vi "Teleop.vi"(10 "Match Info":T4={"Autonomous Elapsed Seconds"=0.0, "TeleOp Elapsed Seconds"=0.0, "Disabled Elapsed Seconds"=0.0, "Visited Autonomous"=FALSE, "Visited TeleOp"=FALSE, "Visited Disabled"=FALSE, "Autonomous Settings"={"Autonomous Style"=enum."Independent", "VI Refnum"=refnum}}, 11 "Call Context":T5) -> ()   [LabVIEW 2015]
doc: "This VI is called for each TeleOp packet received from the DS where the robot is not disabled. It is often used to read from the joysticks and update I/O or to update setpoints for timed control loops. It should complete and return within 20 milliseconds or it may miss DS packets."
uses:
  <vilib>/Rock Robotics/WPI/DriverStation/WPI_DriverStationDerivedRobotMode.ctl
  <vilib>/Rock Robotics/WPI/DriverStation/WPI_DriverStationMatch Info.ctl
  <vilib>/Rock Robotics/WPI/CAN/TalonSRX/WPI_CANTalonSRX_GlobalStatus.ctl
  <vilib>/Rock Robotics/WPI/Solenoid/WPI_SolenoidValue.ctl
  <vilib>/Rock Robotics/WPI/CAN/TalonSRX/WPI_CANTalonSRX_APIFeedbackSelect.ctl
  <vilib>/Rock Robotics/WPI/CAN/TalonSRX/WPI_CANTalonSRX_APIControlMode.ctl
  <vilib>/Rock Robotics/WPI/CAN/TalonSRX/WPI_CANTalonSRX_BrakeOverride.ctl
  <vilib>/Rock Robotics/WPI/Solenoid/WPI_SolenoidGetEnum.vi
  <vilib>/Rock Robotics/WPI/Utilities/WPI_GetSetVariantRefNum.vi
  <vilib>/Rock Robotics/Network Tables/NT Write Boolean Array.vi
  <vilib>/Rock Robotics/Network Tables/NT Write Numeric Array.vi
  <vilib>/Rock Robotics/WPI/Solenoid/WPI_SolenoidSetEnum.vi
  <vilib>/addons/control/pid/pid.llb/PID (DBL).vi
  <vilib>/Rock Robotics/Network Tables/NT Write Boolean.vi
  ADIS16448/ADI MXP IMU/FRC_ADIS16448_IMU.lvlib
  <vilib>/addons/control/pid/NI_PID_pid.lvlib
  Robot Global Data.vi
panel:
  out "Straight Line PID":dbl(graph)
  in  "Straight Line PID gains":T1={"proportional gain (Kc)"=0.15, "integral time (Ti, min)"=0.0, "derivative time (Td, min)"=0.0005} {"proportional gain (Kc)" step=0.001; "integral time (Ti, min)" step=0.001; "derivative time (Td, min)" step=0.001}
  in  "straight line output range":cluster{"output high":dbl, "output low":dbl}={"output high"=1.0, "output low"=-1.0}
  out "SRX Status Right":T2
  in  "Ramp Rate":dbl format="%#_13g"
  in  "I Zone":dbl format="%#_13g"
  in  "F":dbl=0.005212 format="%#_13g"
  in  "D":dbl format="%#_13g"
  in  "I":dbl format="%#_13g"
  in  "P":dbl=0.5 format="%#_13g"
  out "SRX Status Left":T2
  out "Override":bool
  out "Speed":T3(graph)
  # "Drive PID Tuning"
  # "Competition Robot:\n\nP = 0.5\nI = 0\nD = 0\nF = 0.005212\nI Zone = 0\nRamp Rate = 0"
  # "Competition Robot:\nOutput Range\n0.6 / -0.6\n\nP = 30\nI = 0.5\nD = 0"
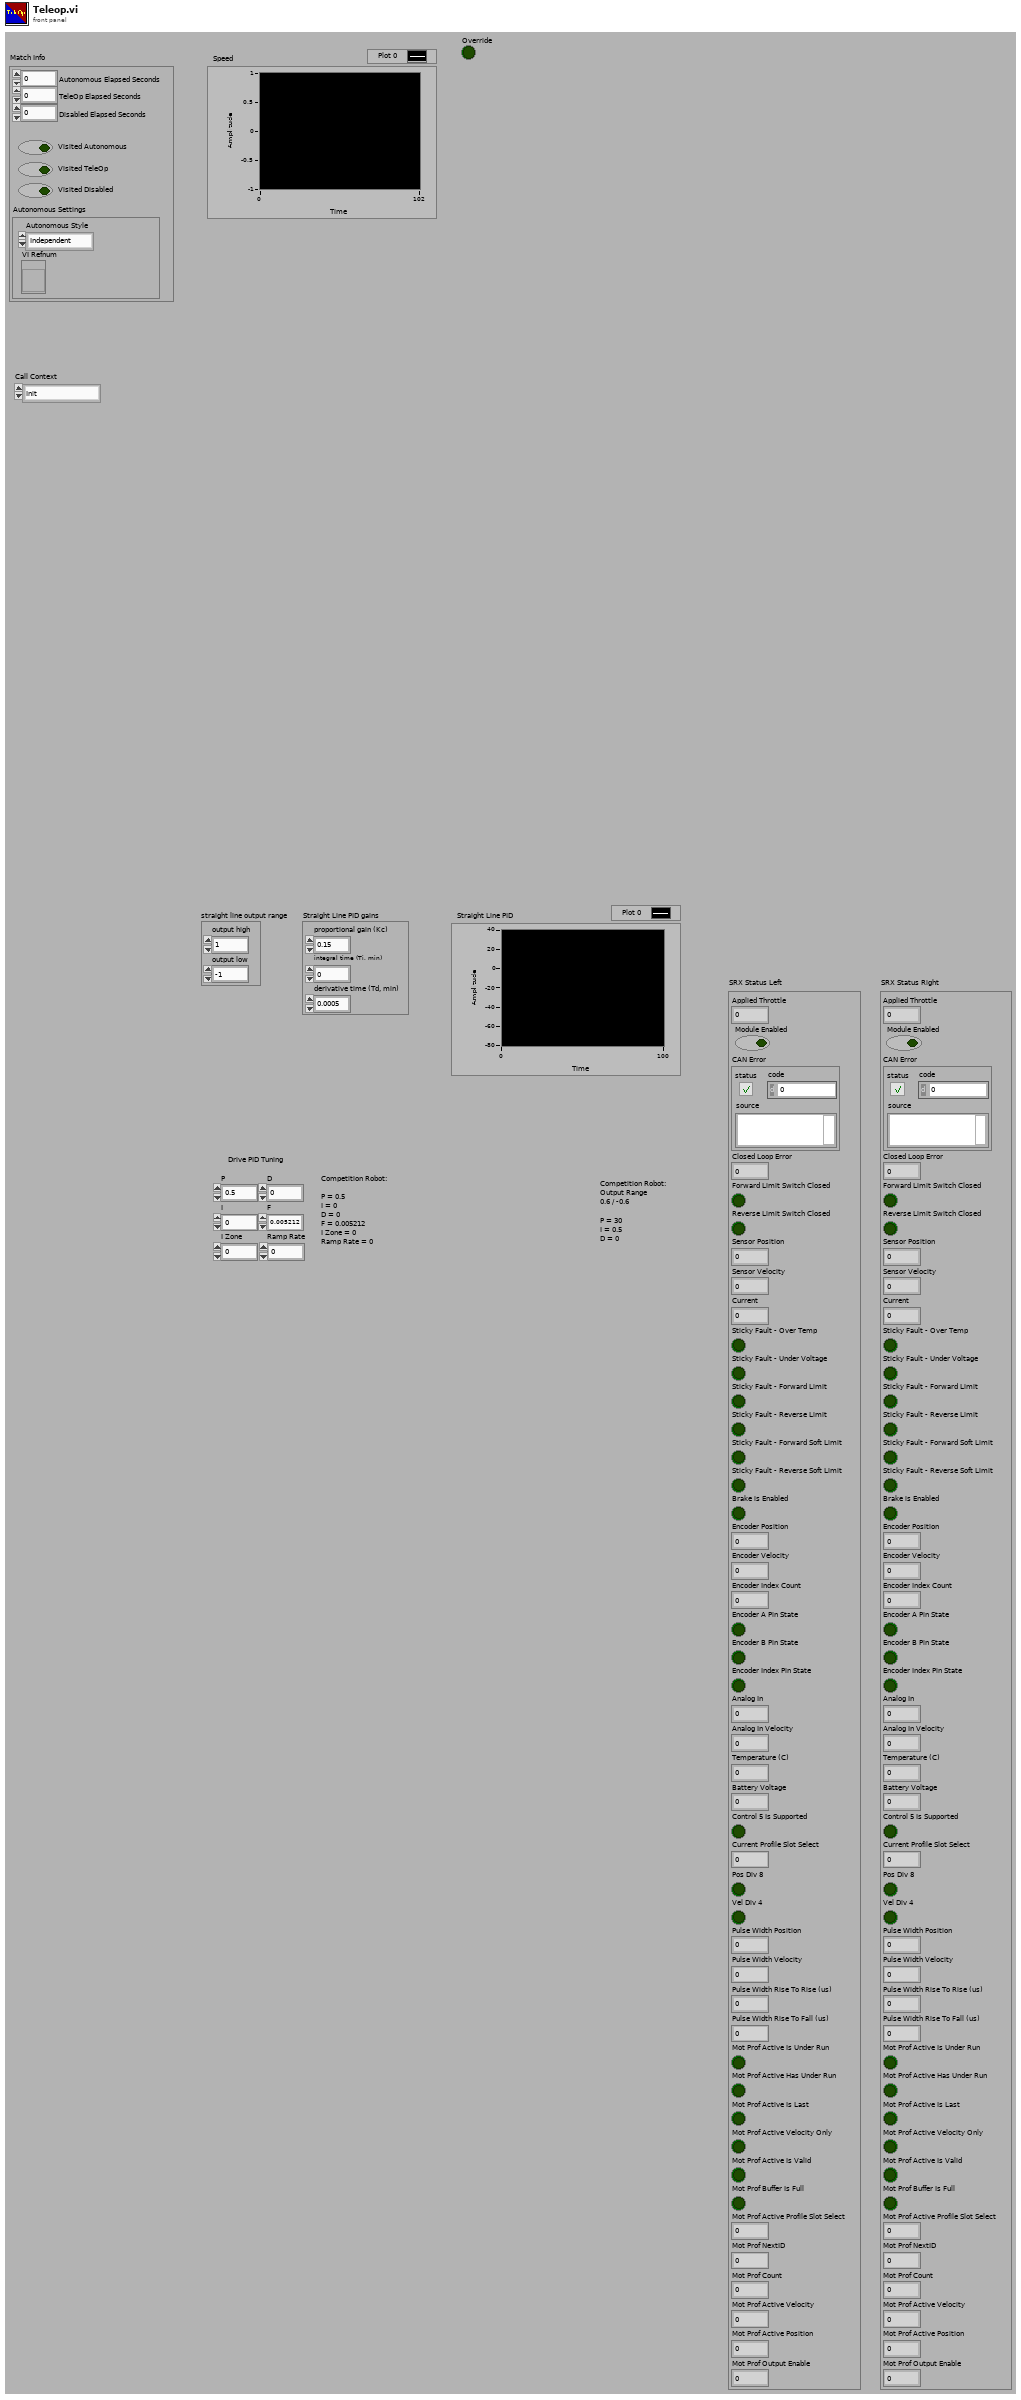
[diagram p1: front panel]
types:
  T1 = cluster{"proportional gain (Kc)":dbl, "integral time (Ti, min)":dbl, "derivative time (Td, min)":dbl}
  T2 = typedef "WPI_CANTalonSRX_GlobalStatus.ctl" = cluster{"Applied Throttle":dbl, "Module Enabled":bool, "CAN Error":errorcluster, "Closed Loop Error":dbl, "Forward Limit Switch Closed":bool, "Reverse Limit Switch Closed":bool, "Sensor Position":dbl, "Sensor Velocity":dbl, "Current":dbl, "Sticky Fault - Over Temp":bool, "Sticky Fault - Under Voltage":bool, "Sticky Fault - Forward Limit":bool, "Sticky Fault - Reverse Limit":bool, "Sticky Fault - Forward Soft Limit":bool, "Sticky Fault - Reverse Soft Limit":bool, "Brake is Enabled":bool, "Encoder Position":dbl, "Encoder Velocity":dbl, "Encoder Index Count":dbl, "Encoder A Pin State":bool, "Encoder B Pin State":bool, "Encoder Index Pin State":bool, "Analog In":dbl, "Analog In Velocity":dbl, "Temperature (C)":dbl, "Battery Voltage":dbl, "Control 5 Is Supported":bool, "Current Profile Slot Select":dbl, "Pos Div 8":bool, "Vel Div 4":bool, "Pulse Width Position":i32, "Pulse Width Velocity":i32, "Pulse Width Rise To Rise (us)":i32, "Pulse Width Rise To Fall (us)":i32, "Mot Prof Active Is Under Run":bool, "Mot Prof Active Has Under Run":bool, "Mot Prof Active Is Last":bool, "Mot Prof Active Velocity Only":bool, "Mot Prof Active Is Valid":bool, "Mot Prof Buffer Is Full":bool, "Mot Prof Active Profile Slot Select":i32, "Mot Prof NextID":i32, "Mot Prof Count":i32, "Mot Prof Active Velocity":dbl, "Mot Prof Active Position":dbl, "Mot Prof Output Enable":i32}
  T3 = cluster{"Left Motor Value":dbl, "Right Motor Value":dbl}
  T4 = typedef "WPI_DriverStationMatch Info.ctl" = cluster{"Autonomous Elapsed Seconds":dbl, "TeleOp Elapsed Seconds":dbl, "Disabled Elapsed Seconds":dbl, "Visited Autonomous":bool, "Visited TeleOp":bool, "Visited Disabled":bool, "Autonomous Settings":cluster{"Autonomous Style":enum16{"Iterative", "Independent"}, "VI Refnum":refnum<vi>}}
  T5 = typedef "WPI_DriverStationDerivedRobotMode.ctl" = enum16{"Init", "Execute", "Stop"}
  T6 = typedef "WPI_SolenoidValue.ctl" = enum16{"Off", "On", "Forward", "Reverse"}
  T7 = typedef "WPI_MotorControlDeviceRef.ctl" = cluster{"DeviceStatus":errorcluster, "Type":T8, "PWM":cluster{"PWM Channel":T9, "DeadBand":T10}, "CAN":cluster{"Device Number":u8, "Control Mode":T11, "Semaphore":T12, "Max Vout":dbl, "TalonSRX Control Mode":T13}, "Invert":bool}
  T8 = typedef "WPI_MotorControlType.ctl" = enum16{"PWM", "CAN", "CANTalonSRX"}
  T9 = typedef "FPGA_DIOPWMChannel.ctl" = enum8{"PWM 0", "PWM 1", "PWM 2", "PWM 3", "PWM 4", "PWM 5", "PWM 6", "PWM 7", "PWM 8", "PWM 9", "PWM MXP 0", "PWM MXP 1", "PWM MXP 2", "PWM MXP 3", "PWM MXP 4", "PWM MXP 5", "PWM MXP 6", "PWM MXP 7", "PWM MXP 8", "PWM MXP 9", "Invalid"}
  T10 = typedef "WPI_PWMDeadband.ctl" = cluster{"Name":string, "maxPositivePwm":i32, "minPositivePwm":i32, "centerPwm":i32, "maxNegativePwm":i32, "minNegativePwm":i32, "angularRange":u16}
  T11 = typedef "WPI_CANJaguar_ControlMode.ctl" = enum8{"Percent VBus", "Current", "Speed", "Position", "Voltage"}
  T12 = typedef "Semaphore RefNum" = refnum<k1>
  T13 = typedef "WPI_CANTalonSRX_APIControlMode.ctl" = enum8{"Percent VBus", "Speed", "Position", "Slave", "Unchanged / Invalid", "Voltage Compensation", "Current", "Motion Profile"}
  T14 = typedef "WPI_JoystickDevRef.ctl" = cluster{"Device":T15}
  T15 = typedef "WPI_JoystickDeviceEnum.ctl" = enum16{"USB 0", "USB 1", "USB 2", "USB 3", "USB 4", "USB 5"}
  T16 = typedef "WPI_SolenoidDevRef.ctl" = cluster{"DevStatus":errorcluster, "Pneumatics Control Module":u8, "Forward Solenoid Channel":T17, "Reverse Solenoid Channel":T17}
  T17 = typedef "WPI_SolenoidChannel.ctl" = enum8{"Solenoid 0", "Solenoid 1", "Solenoid 2", "Solenoid 3", "Solenoid 4", "Solenoid 5", "Solenoid 6", "Solenoid 7", "Invalid"}
  T18 = typedef "WPI_SwitchDevRef.ctl" = cluster{"DevStatus":errorcluster, "DIO Channel":T19, "CntIndex":T20, "Normally Closed":bool}
  T19 = typedef "FPGA_DIOChannel.ctl" = enum8{"DIO 0", "DIO 1", "DIO 2", "DIO 3", "DIO 4", "DIO 5", "DIO 6", "DIO 7", "DIO 8", "DIO 9", "DIO MXP 0", "DIO MXP 1", "DIO MXP 2", "DIO MXP 3", "DIO MXP 4", "DIO MXP 5", "DIO MXP 6", "DIO MXP 7", "DIO MXP 8", "DIO MXP 9", "DIO MXP 10", "DIO MXP 11", "DIO MXP 12", "DIO MXP 13", "DIO MXP 14", "DIO MXP 15", "Invalid"}
  T20 = typedef "FPGA_CounterCtrSystemIndex.ctl" = enum8{"Ctr 0", "Ctr 1", "Ctr 2", "Ctr 3", "Ctr 4", "Ctr 5", "Ctr 6", "Ctr 7", "Invalid"}
  T21 = typedef "FRC_ADIS16448_IMU.lvlib/WPI_IMU_ADIS16448_InterruptDevRef.ctl" = cluster{"ADI IMU DevRef":T22, "InterruptRef":T24}
  T22 = typedef "FRC_ADIS16448_IMU.lvlib/WPI_IMU_ADIS16448_IMUDevRef.ctl" = cluster{"DevStatus":errorcluster, "Handle":i32, "SPI Bus":T23, "Device Found":bool, "Device Ready":bool, "Yaw Axis":enum16{"X", "Y", "Z"}, "AHRS Algorithm":enum16{"Complementary", "Madgwick"}, "Serial":u16, "Lot ID 2":u16, "Lot ID 1":u16, "Product ID":u16}
  T23 = typedef "spi_bus.ctl" = enum16{"SPI On-Board, CS0", "SPI On-Board, CS1", "SPI On-Board, CS2", "SPI On-Board, CS3", "SPI MXP", "Invalid"}
  T24 = typedef "WPI_InterruptRef.ctl" = cluster{"DevStatus":errorcluster, "InterruptIndex":T25}
  T25 = typedef "FPGA_InterruptIndex.ctl" = enum8{"0", "1", "2", "3", "4", "5", "6", "7", "Invalid"}
  T26 = cluster{"X Angle":dbl, "Y Angle":dbl, "Z Angle":dbl}
  T27 = typedef "WPI_CANTalonSRX_APIFeedbackSelect.ctl" = enum16{"Digital Quadrature Encoder", "Analog Potentiometer", "Analog Encoder", "Count on Quad-A (Rising-Edge)", "Count on Quad-A (Falling-Edge)", "CTR Magnetic Enc (Absolute)", "CTR Magnetic Enc (Relative)", "Pulse Width"}
  T28 = typedef "WPI_CANTalonSRX_BrakeOverride.ctl" = enum8{"No Override", "Override to Coast", "Override to Brake"}
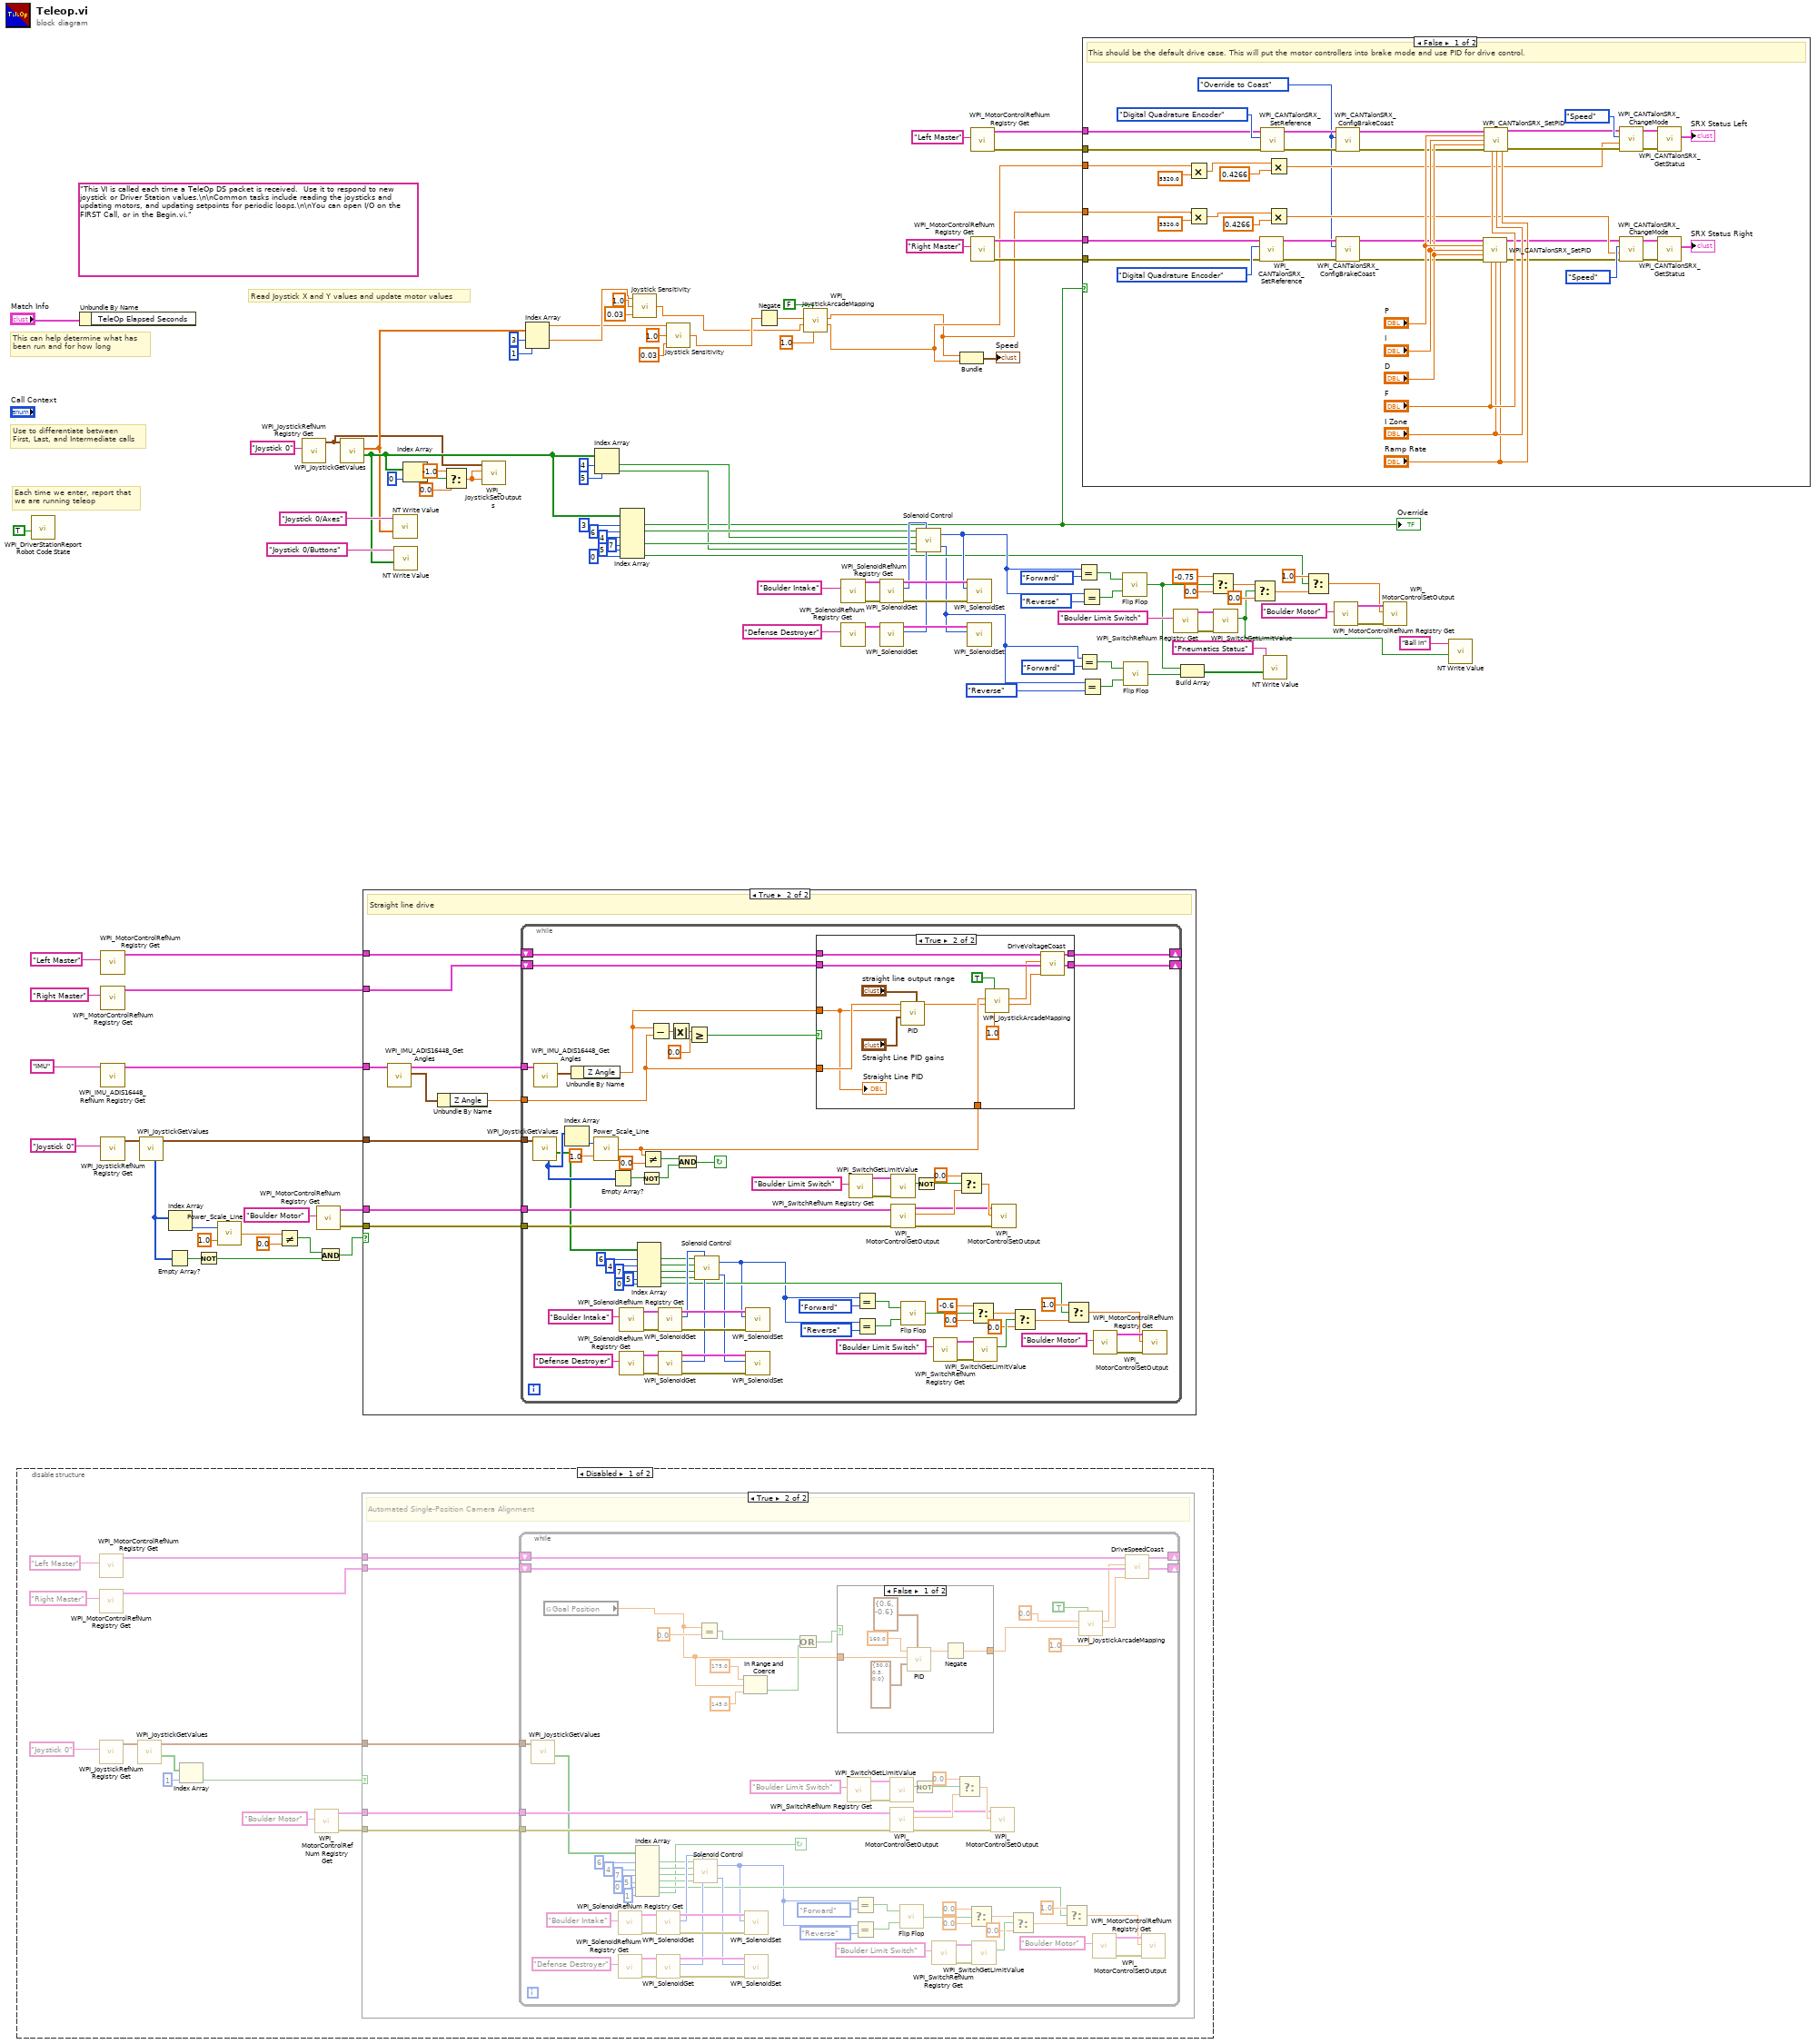
[diagram p0: block diagram]
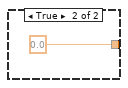
[diagram p3: hidden frame]
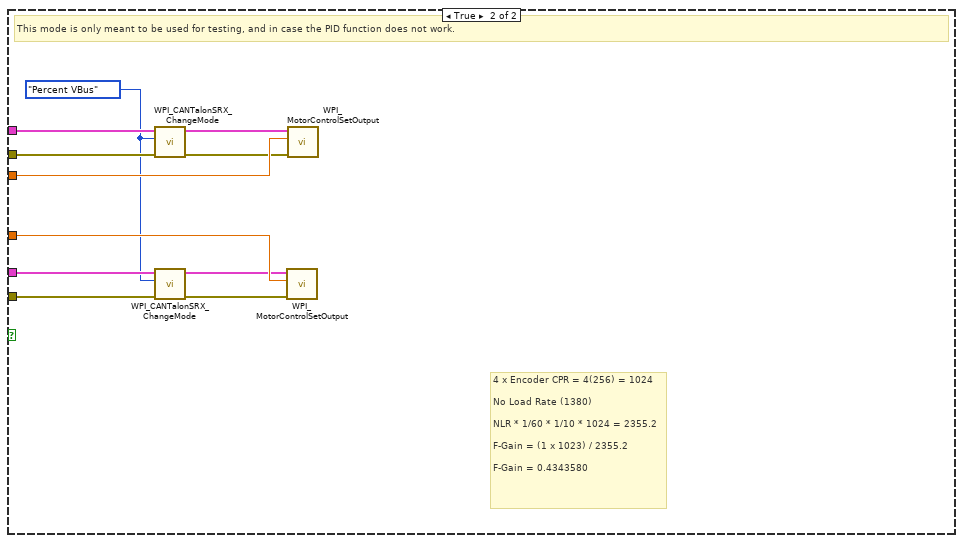
[diagram p5: hidden frame]
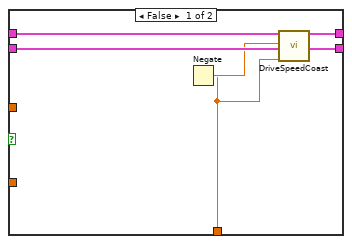
[diagram p7: hidden frame]
diagram:
  (unwired) "This VI is called each time a TeleOp DS packet is received.  Use it to respond to new joystick or Driver Station values.\n\nCommon tasks include reading the joysticks and updating motors, and updating setpoints for periodic loops.\n\nYou can open I/O on the FIRST Call, or in the Begin.vi."
  # "Each time we enter, report that\nwe are running teleop"
  # "Use to differentiate between\nFirst, Last, and Intermediate calls"
  # "This can help determine what has\nbeen run and for how long"
  # "Read Joystick X and Y values and update motor values"
  n1 = disable-structure shown="Disabled" {
    frame Disabled {
      n2 = call <vilib>:"WPI_MotorControlRefNum Registry Get.vi"("refnum name"="Left Master") -> ("MotorControlDevRef"=w111:T7)  [unwired: 9 in, 1 out]
      n3 = call <vilib>:"WPI_MotorControlRefNum Registry Get.vi"("refnum name"="Right Master") -> ("MotorControlDevRef"=w110:T7)  [unwired: 9 in, 1 out]
      n4 = call <vilib>:"WPI_JoystickRefNum Registry Get.vi"("refnum name"="Joystick 0") -> ("JoystickDevRef"=w119:T14)  [unwired: 1 in, 9 out]
      n5 = call <vilib>:"WPI_JoystickGetValues.vi"("JoystickDevRef"=w119) -> ("Buttons"=w114:bool[], "JoystickDevRef"=w118:T14)  [unwired: 6 in, 3 out]
      n6 = Index Array(array=w114, index=1) -> (element=w112:bool)
      n7 = call <vilib>:"WPI_MotorControlRefNum Registry Get.vi"("refnum name"="Boulder Motor") -> ("error out"=w115:errorcluster, "MotorControlDevRef"=w116:T7)  [unwired: 9 in]
      n8 = case shown="True" w112 {
        tunnel: w110 -> [_ w127]
        tunnel: w111 -> [_ w126]
        tunnel: w118 -> [_ w125]
        tunnel: w116 -> [_ w124]
        tunnel: w115 -> [_ w123]
        frame False {
          # "POV not pressed"
        }
        frame True {
          # "Automated Single-Position Camera Alignment"
          n9 = while {
            shift-right: [w202] -> _
            shift-left: w127 -> [w201]
            shift-right: [w203] -> _
            shift-left: w126 -> [w200]
            tunnel: w125 -> [w199]
            tunnel: w124 -> [w191]
            tunnel: w123 -> [w190]
            stop <- w137 continue-if-true
            n10 = call <vilib>:"WPI_JoystickGetValues.vi"("JoystickDevRef"=w199) -> ("Buttons"=w145:bool[])  [unwired: 6 in, 4 out]
            n11 = global read "Robot Global Data.vi" "Goal Position"() -> (w128:dbl)
            n12 = call <vilib>:"WPI_SolenoidRefNum Registry Get.vi"("refnum name"="Boulder Intake") -> ("error out"=w162:errorcluster, "SolenoidDevRef"=w165:T16)  [unwired: 9 in]
            n13 = call <vilib>:"WPI_SolenoidRefNum Registry Get.vi"("refnum name"="Defense Destroyer") -> ("error out"=w160:errorcluster, "SolenoidDevRef"=w161:T16)  [unwired: 9 in]
            n14 = Index Array(array=w145, index #1=6 ("index"), index #2=4 ("index"), index #3=7 ("index"), index #4=5 ("index"), index #5=0 ("index"), index #6=1 ("index")) -> (element #1=w150:bool, element #2=w149:bool, element #3=w148:bool, element #4=w147:bool, element #5=w146:bool, element #6=w137:bool)
            n15 = call-poly <vilib>:"WPI_SolenoidGet.vi"("error in (no error)"=w162, "SolenoidDevRef"=w165) -> ("error out"=w163:errorcluster, "Value"=w157:T6, "SolenoidDevRef"=w164:T16)  [unwired: 7 in]
            n16 = call-poly <vilib>:"WPI_SolenoidGet.vi"("error in (no error)"=w160, "SolenoidDevRef"=w161) -> ("error out"=w158:errorcluster, "Value"=w156:T6, "SolenoidDevRef"=w159:T16)  [unwired: 7 in]
            n17 = call "Solenoid Control.vi"("Defense Get"=w156, "Ball Get"=w157, "Both Down"=w147, "Both Up"=w148, "Ball Down"=w149, "Ball Up"=w150) -> ("Defense Output"=w155:T6, "Ball Output"=w144:T6)
            n18 = Equal?(x=w128, y=0.0) -> (x = y?=w131:bool)
            n19 = In Range and Coerce(upper limit=175.0, x=w128, lower limit=145.0) -> (In Range?=w130:bool)  [unwired: 1 out]
            n20 = call-poly <vilib>:"WPI_SolenoidSet.vi"("error in (no error)"=w163, "Value"=w144, "SolenoidDevRef"=w164) -> ()  [unwired: 7 in, 2 out]
            n21 = call-poly <vilib>:"WPI_SolenoidSet.vi"("error in (no error)"=w158, "Value"=w155, "SolenoidDevRef"=w159) -> ()  [unwired: 7 in, 2 out]
            n22 = Or(x=w131, y=w130) -> (x .or. y?=w132:bool)
            n23 = case shown="False" w132 {
              tunnel: w128 -> [w209 _]
              tunnel: [w207 0.0 ("output")] -> w135
              frame False {
                n24 = call-poly <vilib>:"PID.vi"("output range"=cluster{"output high":dbl, "output low":dbl} {"output high"=0.6, "output low"=-0.6}, "PID gains"=T1 {"proportional gain (Kc)"=30.0, "integral time (Ti, min)"=0.5, "derivative time (Td, min)"=0.0}, "process variable"=w209, "setpoint"=160.0) -> ("output"=w208:dbl)  [unwired: 6 in, 1 out]
                n25 = Negate(x=w208) -> (-x=w207:dbl)
              }
              frame True {
              }
            }
            n26 = call <vilib>:"WPI_SwitchRefNum Registry Get.vi"("refnum name"="Boulder Limit Switch") -> ("error out"=w198:errorcluster, "SwitchDevRef"=w197:T18)  [unwired: 9 in]
            n27 = Equal?(x=w144, y=WPI_SolenoidValue."Forward" ("Ball Output")) -> (x = y?=w153:bool)
            n28 = Equal?(x=w144, y=WPI_SolenoidValue."Reverse") -> (x = y?=w151:bool)
            n29 = call <vilib>:"WPI_SwitchGetLimitValue.vi"("error in (no error)"=w198, "SwitchDevRef"=w197) -> ("Switch Pressed"=w188:bool)  [unwired: 7 in, 2 out]
            n30 = call <vilib>:"WPI_MotorControlGetOutput.vi"("error in (no error)"=w190, "MotorControlDevRef"=w191) -> ("error out"=w192:errorcluster, "Output"=w194:dbl, "MotorControlDevRef"=w193:T7)  [unwired: 7 in]
            n31 = call "Flip Flop.vi"("Reset"=w151, "Value to be latched"=w153) -> ("Indicator"=w169:bool)
            n32 = Not(x=w188) -> (.not. x?=w189:bool)
            n33 = call <vilib>:"WPI_SwitchRefNum Registry Get.vi"("refnum name"="Boulder Limit Switch") -> ("error out"=w179:errorcluster, "SwitchDevRef"=w178:T18)  [unwired: 9 in]
            n34 = Select(t=0.0, s=w189, f=w194) -> (s? t:f=w195:dbl)
            n35 = Select(t=0.0, s=w169, f=0.0) -> (s? t:f=w173:dbl)
            n36 = call <vilib>:"WPI_SwitchGetLimitValue.vi"("error in (no error)"=w179, "SwitchDevRef"=w178) -> ("Switch Pressed"=w175:bool)  [unwired: 7 in, 2 out]
            n37 = call <vilib>:"WPI_MotorControlSetOutput.vi"("error in (no error)"=w192, "Output"=w195, "MotorControlDevRef"=w193) -> ()  [unwired: 6 in, 3 out]
            n38 = Select(t=w173, s=w175, f=0.0) -> (s? t:f=w172:dbl)
            n39 = Select(t=1.0, s=w146, f=w172) -> (s? t:f=w171:dbl)
            n40 = call <vilib>:"WPI_JoystickArcadeMapping.vi"("Max Output"=1.0, "Square Inputs"=TRUE, "Y axis value"=w135, "X axis value"=0.0 ("Power Input")) -> ("Right Motor Value"=w140:dbl, "Left Motor Value"=w139:dbl)  [unwired: 6 in]
            n41 = call <vilib>:"WPI_MotorControlRefNum Registry Get.vi"("refnum name"="Boulder Motor") -> ("error out"=w181:errorcluster, "MotorControlDevRef"=w182:T7)  [unwired: 9 in]
            n42 = call "DriveSpeedCoast.vi"("Left Motor"=w200, "Left Stick"=w139, "Right Motor"=w201, "Right Stick"=w140) -> ("Left Motor Out"=w203:T7, "Right Motor Out"=w202:T7)  [unwired: 10 in, 4 out]
            n43 = call <vilib>:"WPI_MotorControlSetOutput.vi"("error in (no error)"=w181, "Output"=w171, "MotorControlDevRef"=w182) -> ()  [unwired: 6 in, 3 out]
          }
        }
      }
    }
    frame Enabled {
    }
  }
  n44 = call <vilib>:"WPI_DriverStationReport Robot Code State.vi"("TeleOp"=TRUE ("Autonomous")) -> ()  [unwired: 10 in, 1 out]
  n45 = Unbundle By Name("Match Info") -> ()  [unwired: 1 out]
  n46 = call <vilib>:"WPI_MotorControlRefNum Registry Get.vi"("refnum name"="Left Master") -> ("MotorControlDevRef"=w5:T7)  [unwired: 9 in, 1 out]
  n47 = call <vilib>:"WPI_MotorControlRefNum Registry Get.vi"("refnum name"="Right Master") -> ("MotorControlDevRef"=w4:T7)  [unwired: 9 in, 1 out]
  n48 = call "WPI_IMU_ADIS16448_RefNum Registry Get.vi"("refnum name"="IMU") -> ("ADI IMU Interrupt DevRef"=w24:T21)  [unwired: 9 in, 1 out]
  n49 = call <vilib>:"WPI_JoystickRefNum Registry Get.vi"("refnum name"="Joystick 0") -> ("JoystickDevRef"=w21:T14)  [unwired: 1 in, 9 out]
  n50 = call <vilib>:"WPI_JoystickGetValues.vi"("JoystickDevRef"=w21) -> ("JoystickDevRef"=w20:T14, "POVs"=w19:i16[])  [unwired: 6 in, 3 out]
  n51 = Empty Array?(array=w19) -> (empty?=w18:bool)
  n52 = Index Array(array=w19) -> (element=w23:i16)  [unwired: 1 in]
  n53 = Not(x=w18) -> (.not. x?=w17:bool)
  n54 = call "Power_Scale_Line.vi"("Power Input"=1.0, "POV"=w23) -> ("Power Output"=w25:dbl)
  n55 = Not Equal?(x=w25, y=0.0) -> (x != y?=w16:bool)
  n56 = call <vilib>:"WPI_JoystickRefNum Registry Get.vi"("refnum name"="Joystick 0") -> ("JoystickDevRef"=w31:T14)  [unwired: 1 in, 9 out]
  n57 = call <vilib>:"WPI_MotorControlRefNum Registry Get.vi"("refnum name"="Boulder Motor") -> ("error out"=w12:errorcluster, "MotorControlDevRef"=w13:T7)  [unwired: 9 in]
  n58 = And(x=w16, y=w17) -> (x .and. y?=w15:bool)
  n59 = call <vilib>:"WPI_JoystickGetValues.vi"("JoystickDevRef"=w31) -> ("Buttons"=w38:bool[], "Axes"=w32:dbl[])  [unwired: 6 in, 3 out]
  n60 = case shown="True" w15 {
    tunnel: w24 -> [_ w211]
    tunnel: w20 -> [_ w218]
    tunnel: w13 -> [_ w215]
    tunnel: w12 -> [_ w214]
    tunnel: w5 -> [_ w213]
    tunnel: w4 -> [_ w212]
    frame False {
      # "POV not pressed"
    }
    frame True {
      # "Straight line drive"
      n61 = call "WPI_IMU_ADIS16448_Get Angles.vi"("ADI IMU Interrupt DevRef"=w211) -> ("IMU Angles Out"=w216:T26, "ADI IMU Interrupt DevRef Out"=w217:T21)  [unwired: 7 in, 2 out]
      n62 = Unbundle By Name(w216) -> ("Z Angle"=w219:dbl)
      n63 = while {
        tunnel: w217 -> [w278]
        tunnel: w219 -> [w289]
        shift-right: [w293] -> _
        shift-left: w212 -> [w292]
        shift-right: [w294] -> _
        shift-left: w213 -> [w291]
        tunnel: w218 -> [w286]
        tunnel: w215 -> [w269]
        tunnel: w214 -> [w268]
        stop <- w282 continue-if-true
        n64 = call <vilib>:"WPI_JoystickGetValues.vi"("JoystickDevRef"=w286) -> ("Buttons"=w222:bool[], "POVs"=w281:i16[])  [unwired: 6 in, 3 out]
        n65 = call "WPI_IMU_ADIS16448_Get Angles.vi"("ADI IMU Interrupt DevRef"=w278) -> ("IMU Angles Out"=w277:T26)  [unwired: 7 in, 3 out]
        n66 = Index Array(array=w281) -> (element=w295:i16)  [unwired: 1 in]
        n67 = Unbundle By Name(w277) -> ("Z Angle"=w267:dbl)
        n68 = call "Power_Scale_Line.vi"("Power Input"=1.0, "POV"=w295) -> ("Power Output"=w290:dbl)
        n69 = Empty Array?(array=w281) -> (empty?=w285:bool)
        n70 = call <vilib>:"WPI_SolenoidRefNum Registry Get.vi"("refnum name"="Boulder Intake") -> ("error out"=w239:errorcluster, "SolenoidDevRef"=w242:T16)  [unwired: 9 in]
        n71 = call <vilib>:"WPI_SolenoidRefNum Registry Get.vi"("refnum name"="Defense Destroyer") -> ("error out"=w237:errorcluster, "SolenoidDevRef"=w238:T16)  [unwired: 9 in]
        n72 = Index Array(array=w222, index #1=6 ("index"), index #2=4 ("index"), index #3=7 ("index"), index #4=5 ("index"), index #5=0 ("index")) -> (element #1=w227:bool, element #2=w226:bool, element #3=w225:bool, element #4=w224:bool, element #5=w223:bool)
        n73 = Not(x=w285) -> (.not. x?=w284:bool)
        n74 = Not Equal?(x=w290, y=0.0) -> (x != y?=w283:bool)
        n75 = Subtract(x=w267, y=w289) -> (x-y=w280:dbl)
        n76 = call-poly <vilib>:"WPI_SolenoidGet.vi"("error in (no error)"=w239, "SolenoidDevRef"=w242) -> ("error out"=w240:errorcluster, "Value"=w234:T6, "SolenoidDevRef"=w241:T16)  [unwired: 7 in]
        n77 = call-poly <vilib>:"WPI_SolenoidGet.vi"("error in (no error)"=w237, "SolenoidDevRef"=w238) -> ("error out"=w235:errorcluster, "Value"=w233:T6, "SolenoidDevRef"=w236:T16)  [unwired: 7 in]
        n78 = Absolute Value(x=w280) -> (abs(x)=w279:dbl)
        n79 = And(x=w283, y=w284) -> (x .and. y?=w282:bool)
        n80 = Greater Or Equal?(x=w279, y=0.0 ("within")) -> (x >= y?=w287:bool)
        n81 = call "Solenoid Control.vi"("Defense Get"=w233, "Ball Get"=w234, "Both Down"=w224, "Both Up"=w225, "Ball Down"=w226, "Ball Up"=w227) -> ("Defense Output"=w232:T6, "Ball Output"=w221:T6)
        n82 = call-poly <vilib>:"WPI_SolenoidSet.vi"("error in (no error)"=w240, "Value"=w221, "SolenoidDevRef"=w241) -> ()  [unwired: 7 in, 2 out]
        n83 = call-poly <vilib>:"WPI_SolenoidSet.vi"("error in (no error)"=w235, "Value"=w232, "SolenoidDevRef"=w236) -> ()  [unwired: 7 in, 2 out]
        n84 = case shown="True" w287 {
          tunnel: [w302 w308] -> w294
          tunnel: [w301 w309] -> w293
          tunnel: w292 -> [w300 w311]
          tunnel: w291 -> [w303 w312]
          tunnel: w290 -> [w298 w306]
          tunnel: w267 -> [_ w304]
          tunnel: w289 -> [_ w317]
          frame False {
            n85 = Negate(x=w298) -> (-x=w299:dbl)
            n86 = call "DriveSpeedCoast.vi"("Left Motor"=w303, "Left Stick"=w299, "Right Motor"=w300, "Right Stick"=w298) -> ("Left Motor Out"=w302:T7, "Right Motor Out"=w301:T7)  [unwired: 10 in, 4 out]
          }
          frame True {
            n87 = call-poly <vilib>:"PID.vi"("output range"="straight line output range", "PID gains"="Straight Line PID gains", "process variable"=w304, "setpoint"=w317) -> ("output"=w305:dbl)  [unwired: 6 in, 1 out]
            n88 = call <vilib>:"WPI_JoystickArcadeMapping.vi"("Max Output"=1.0, "Square Inputs"=TRUE, "Y axis value"=w305, "X axis value"=w306) -> ("Right Motor Value"=w310:dbl, "Left Motor Value"=w307:dbl)  [unwired: 6 in]
            n89 = call "DriveVoltageCoast.vi"("Left Motor"=w312, "Left Stick"=w307, "Right Motor"=w311, "Right Stick"=w310) -> ("Left Motor Out"=w308:T7, "Right Motor Out"=w309:T7)  [unwired: 12 in, 2 out]
            "Straight Line PID" <- w304
          }
        }
        n90 = call <vilib>:"WPI_SwitchRefNum Registry Get.vi"("refnum name"="Boulder Limit Switch") -> ("error out"=w276:errorcluster, "SwitchDevRef"=w275:T18)  [unwired: 9 in]
        n91 = Equal?(x=w221, y=WPI_SolenoidValue."Forward" ("Ball Output")) -> (x = y?=w230:bool)
        n92 = Equal?(x=w221, y=WPI_SolenoidValue."Reverse") -> (x = y?=w228:bool)
        n93 = call <vilib>:"WPI_SwitchGetLimitValue.vi"("error in (no error)"=w276, "SwitchDevRef"=w275) -> ("Switch Pressed"=w265:bool)  [unwired: 7 in, 2 out]
        n94 = call <vilib>:"WPI_MotorControlGetOutput.vi"("error in (no error)"=w268, "MotorControlDevRef"=w269) -> ("error out"=w270:errorcluster, "Output"=w272:dbl, "MotorControlDevRef"=w271:T7)  [unwired: 7 in]
        n95 = call "Flip Flop.vi"("Reset"=w228, "Value to be latched"=w230) -> ("Indicator"=w246:bool)
        n96 = Not(x=w265) -> (.not. x?=w266:bool)
        n97 = call <vilib>:"WPI_SwitchRefNum Registry Get.vi"("refnum name"="Boulder Limit Switch") -> ("error out"=w256:errorcluster, "SwitchDevRef"=w255:T18)  [unwired: 9 in]
        n98 = Select(t=0.0, s=w266, f=w272) -> (s? t:f=w273:dbl)
        n99 = Select(t=-0.6, s=w246, f=0.0) -> (s? t:f=w250:dbl)
        n100 = call <vilib>:"WPI_SwitchGetLimitValue.vi"("error in (no error)"=w256, "SwitchDevRef"=w255) -> ("Switch Pressed"=w252:bool)  [unwired: 7 in, 2 out]
        n101 = call <vilib>:"WPI_MotorControlSetOutput.vi"("error in (no error)"=w270, "Output"=w273, "MotorControlDevRef"=w271) -> ()  [unwired: 6 in, 3 out]
        n102 = Select(t=w250, s=w252, f=0.0) -> (s? t:f=w249:dbl)
        n103 = Select(t=1.0, s=w223, f=w249) -> (s? t:f=w248:dbl)
        n104 = call <vilib>:"WPI_MotorControlRefNum Registry Get.vi"("refnum name"="Boulder Motor") -> ("error out"=w258:errorcluster, "MotorControlDevRef"=w259:T7)  [unwired: 9 in]
        n105 = call <vilib>:"WPI_MotorControlSetOutput.vi"("error in (no error)"=w258, "Output"=w248, "MotorControlDevRef"=w259) -> ()  [unwired: 6 in, 3 out]
      }
    }
  }
  n106 = call-poly <vilib>:"NT Write Value.vi"("Numeric Array"=w32, "Name"="Joystick 0/Axes") -> ()  [unwired: 9 in, 1 out]
  n107 = call-poly <vilib>:"NT Write Value.vi"("Boolean Array"=w38, "Name"="Joystick 0/Buttons") -> ()  [unwired: 9 in, 1 out]
  n108 = Index Array(array=w38, index=0) -> (element=w36:bool)
  n109 = Select(t=-1.0, s=w36, f=0.0) -> (s? t:f=w33:dbl)
  n110 = call <vilib>:"WPI_JoystickSetOutputs.vi"("Right Rumble"=w33, "Left Rumble"=w33, "JoystickDevRef"=w31) -> ()  [unwired: 7 in, 2 out]
  n111 = Index Array(array=w32, index #1=3 ("index"), index #2=1 ("index")) -> (element #1=w44:dbl, element #2=w43:dbl)
  n112 = Index Array(array=w38, index #1=4 ("index"), index #2=5 ("index")) -> (element #1=w55:bool, element #2=w54:bool)
  n113 = Index Array(array=w38, index #1=3 ("index"), index #2=6 ("index"), index #3=4 ("index"), index #4=7 ("index"), index #5=5 ("index"), index #6=0 ("index")) -> (element #1=w3:bool, element #2=w70:bool, element #4=w69:bool, element #6=w68:bool)  [unwired: 2 out]
  "Override" <- w3
  n114 = call "Joystick Sensitivity.vi"("B"=0.03, "A"=1.0, "X"=w44) -> ("Y"=w41:dbl)
  n115 = call "Joystick Sensitivity.vi"("B"=0.03, "A"=1.0, "X"=w43) -> ("Y"=w42:dbl)
  n116 = Negate(x=w42) -> (-x=w51:dbl)
  n117 = call <vilib>:"WPI_JoystickArcadeMapping.vi"("Max Output"=1.0, "Square Inputs"=FALSE, "Y axis value"=w41, "X axis value"=w51) -> ("Right Motor Value"=w7:dbl, "Left Motor Value"=w6:dbl)  [unwired: 6 in]
  n118 = call <vilib>:"WPI_SolenoidRefNum Registry Get.vi"("refnum name"="Boulder Intake") -> ("error out"=w80:errorcluster, "SolenoidDevRef"=w83:T16)  [unwired: 9 in]
  n119 = call <vilib>:"WPI_SolenoidRefNum Registry Get.vi"("refnum name"="Defense Destroyer") -> ("SolenoidDevRef"=w79:T16)  [unwired: 9 in, 1 out]
  n120 = call-poly <vilib>:"WPI_SolenoidGet.vi"("error in (no error)"=w80, "SolenoidDevRef"=w83) -> ("error out"=w81:errorcluster, "Value"=w77:T6, "SolenoidDevRef"=w82:T16)  [unwired: 7 in]
  n121 = call-poly <vilib>:"WPI_SolenoidGet.vi"("SolenoidDevRef"=w79) -> ("Value"=w76:T6, "SolenoidDevRef"=w78:T16)  [unwired: 8 in, 1 out]
  n122 = call "Solenoid Control.vi"("Defense Get"=w76, "Ball Get"=w77, "Both Down"=w54, "Both Up"=w69, "Ball Down"=w55, "Ball Up"=w70) -> ("Defense Output"=w60:T6, "Ball Output"=w71:T6)
  n123 = Bundle("Left Motor Value"=w6, "Right Motor Value"=w7) -> (→"Speed":T3)  [unwired: 1 in]
  n124 = call-poly <vilib>:"WPI_SolenoidSet.vi"("error in (no error)"=w81, "Value"=w71, "SolenoidDevRef"=w82) -> ()  [unwired: 7 in, 2 out]
  n125 = call-poly <vilib>:"WPI_SolenoidSet.vi"("Value"=w60, "SolenoidDevRef"=w78) -> ()  [unwired: 8 in, 2 out]
  n126 = call <vilib>:"WPI_MotorControlRefNum Registry Get.vi"("refnum name"="Left Master") -> ("error out"=w10:errorcluster, "MotorControlDevRef"=w11:T7)  [unwired: 9 in]
  n127 = call <vilib>:"WPI_MotorControlRefNum Registry Get.vi"("refnum name"="Right Master") -> ("error out"=w8:errorcluster, "MotorControlDevRef"=w9:T7)  [unwired: 9 in]
  n128 = Equal?(x=w71, y=WPI_SolenoidValue."Forward" ("Ball Output")) -> (x = y?=w74:bool)
  n129 = Equal?(x=w60, y=WPI_SolenoidValue."Forward" ("Ball Output")) -> (x = y?=w63:bool)
  n130 = Equal?(x=w71, y=WPI_SolenoidValue."Reverse") -> (x = y?=w72:bool)
  n131 = Equal?(x=w60, y=WPI_SolenoidValue."Reverse") -> (x = y?=w61:bool)
  n132 = case shown="False" w3 {
    tunnel: w11 -> [w338 w365]
    tunnel: w10 -> [w337 w364]
    tunnel: w9 -> [w336 w369]
    tunnel: w8 -> [w335 w368]
    tunnel: w7 -> [w334 w371]
    tunnel: w6 -> [w333 w370]
    frame False {
      w325 = WPI_CANTalonSRX_BrakeOverride."Override to Coast" ("Brake / Coast Mode")
      # "This should be the default drive case. This will put the motor controllers into brake mode and use PID for drive control."
      n133 = Multiply(x=w334, y=5320.0) -> (x*y=w347:dbl)
      n134 = Multiply(x=w333, y=5320.0) -> (x*y=w350:dbl)
      n135 = call <vilib>:"WPI_CANTalonSRX_SetReference.vi"("error in (no error)"=w335, "Feedback Reference"=WPI_CANTalonSRX_APIFeedbackSelect."Digital Quadrature Encoder", "CAN Talon SRX Ref"=w336) -> ("error out"=w326:errorcluster, "CAN Talon SRX Ref"=w327:T7)  [unwired: 7 in]
      n136 = call <vilib>:"WPI_CANTalonSRX_SetReference.vi"("error in (no error)"=w337, "Feedback Reference"=WPI_CANTalonSRX_APIFeedbackSelect."Digital Quadrature Encoder", "CAN Talon SRX Ref"=w338) -> ("error out"=w329:errorcluster, "CAN Talon SRX Ref"=w328:T7)  [unwired: 7 in]
      n137 = Multiply(x=w347, y=0.4266) -> (x*y=w342:dbl)
      n138 = Multiply(x=w350, y=0.4266) -> (x*y=w341:dbl)
      n139 = call <vilib>:"WPI_CANTalonSRX_ConfigBrakeCoast.vi"("error in (no error)"=w329, "Brake / Coast Mode"=w325, "CAN Talon SRX Ref"=w328) -> ("error out"=w323:errorcluster, "CAN Talon SRX Ref"=w324:T7)  [unwired: 7 in]
      n140 = call <vilib>:"WPI_CANTalonSRX_ConfigBrakeCoast.vi"("error in (no error)"=w326, "Brake / Coast Mode"=w325, "CAN Talon SRX Ref"=w327) -> ("error out"=w321:errorcluster, "CAN Talon SRX Ref"=w322:T7)  [unwired: 7 in]
      n141 = call <vilib>:"WPI_CANTalonSRX_SetPID.vi"("CAN Talon SRX Ref"=w322, "P"="P", "I"="I", "D"="D", "error in (no error)"=w321, "F"="F", "I Zone"="I Zone", "Ramp Rate"="Ramp Rate") -> ("CAN Talon SRX Ref"=w340:T7, "error out"=w339:errorcluster)  [unwired: 6 in]
      n142 = call <vilib>:"WPI_CANTalonSRX_SetPID.vi"("CAN Talon SRX Ref"=w324, "P"="P", "I"="I", "D"="D", "error in (no error)"=w323, "F"="F", "I Zone"="I Zone", "Ramp Rate"="Ramp Rate") -> ("CAN Talon SRX Ref"=w343:T7, "error out"=w344:errorcluster)  [unwired: 6 in]
      n143 = call <vilib>:"WPI_CANTalonSRX_ChangeMode.vi"("error in (no error)"=w344, "Output"=w342, "Control Mode"=WPI_CANTalonSRX_APIControlMode."Speed", "CAN Talon SRX Ref"=w343) -> ("error out"=w332:errorcluster, "CAN Talon SRX Ref"=w331:T7)  [unwired: 6 in]
      n144 = call <vilib>:"WPI_CANTalonSRX_ChangeMode.vi"("error in (no error)"=w339, "Output"=w341, "Control Mode"=WPI_CANTalonSRX_APIControlMode."Speed", "CAN Talon SRX Ref"=w340) -> ("error out"=w320:errorcluster, "CAN Talon SRX Ref"=w319:T7)  [unwired: 6 in]
      n145 = call <vilib>:"WPI_CANTalonSRX_GetStatus.vi"("error in (no error)"=w332, "CAN Talon SRX Ref"=w331) -> ("Talon SRX Status"=→"SRX Status Left":T2)  [unwired: 7 in, 2 out]
      n146 = call <vilib>:"WPI_CANTalonSRX_GetStatus.vi"("error in (no error)"=w320, "CAN Talon SRX Ref"=w319) -> ("Talon SRX Status"=→"SRX Status Right":T2)  [unwired: 7 in, 2 out]
    }
    frame True {
      w361 = WPI_CANTalonSRX_APIControlMode."Percent VBus" ("Control Mode")
      # "4 x Encoder CPR = 4(256) = 1024\n\nNo Load Rate (1380)\n\nNLR * 1/60 * 1/10 * 1024 = 2355.2\n\nF-Gain = (1 x 1023) / 2355.2\n\nF-Gain = 0.4343580"
      # "This mode is only meant to be used for testing, and in case the PID function does not work."
      n147 = call <vilib>:"WPI_CANTalonSRX_ChangeMode.vi"("error in (no error)"=w364, "Control Mode"=w361, "CAN Talon SRX Ref"=w365) -> ("error out"=w362:errorcluster, "CAN Talon SRX Ref"=w363:T7)  [unwired: 7 in]
      n148 = call <vilib>:"WPI_CANTalonSRX_ChangeMode.vi"("error in (no error)"=w368, "Control Mode"=w361, "CAN Talon SRX Ref"=w369) -> ("error out"=w366:errorcluster, "CAN Talon SRX Ref"=w367:T7)  [unwired: 7 in]
      n149 = call <vilib>:"WPI_MotorControlSetOutput.vi"("error in (no error)"=w366, "Output"=w370, "MotorControlDevRef"=w367) -> ()  [unwired: 6 in, 3 out]
      n150 = call <vilib>:"WPI_MotorControlSetOutput.vi"("error in (no error)"=w362, "Output"=w371, "MotorControlDevRef"=w363) -> ()  [unwired: 6 in, 3 out]
    }
  }
  n151 = call "Flip Flop.vi"("Reset"=w72, "Value to be latched"=w74) -> ("Indicator"=w58:bool)
  n152 = call "Flip Flop.vi"("Reset"=w61, "Value to be latched"=w63) -> ("Indicator"=w57:bool)
  n153 = call <vilib>:"WPI_SwitchRefNum Registry Get.vi"("refnum name"="Boulder Limit Switch") -> ("error out"=w94:errorcluster, "SwitchDevRef"=w93:T18)  [unwired: 9 in]
  n154 = Build Array(w58, w57) -> (w56:bool[])
  n155 = Select(t=-0.75, s=w58, f=0.0) -> (s? t:f=w89:dbl)
  n156 = call <vilib>:"WPI_SwitchGetLimitValue.vi"("error in (no error)"=w94, "SwitchDevRef"=w93) -> ("Switch Pressed"=w2:bool)  [unwired: 7 in, 2 out]
  n157 = Select(t=w89, s=w2, f=0.0) -> (s? t:f=w88:dbl)
  n158 = call-poly <vilib>:"NT Write Value.vi"("Boolean Array"=w56, "Name"="Pneumatics Status") -> ()  [unwired: 9 in, 1 out]
  n159 = Select(t=1.0, s=w68, f=w88) -> (s? t:f=w87:dbl)
  n160 = call <vilib>:"WPI_MotorControlRefNum Registry Get.vi"("refnum name"="Boulder Motor") -> ("error out"=w96:errorcluster, "MotorControlDevRef"=w97:T7)  [unwired: 9 in]
  n161 = call <vilib>:"WPI_MotorControlSetOutput.vi"("error in (no error)"=w96, "Output"=w87, "MotorControlDevRef"=w97) -> ()  [unwired: 6 in, 3 out]
  n162 = call-poly <vilib>:"NT Write Value.vi"("Boolean"=w2, "Name"="Ball in") -> ()  [unwired: 9 in, 1 out]
